vi "moveXYZ.vi"() -> ()   [LabVIEW 2014]
panel:
  in  "Z-Position":dbl=30.0
  in  "Y-Position":dbl
  in  "X-Position":dbl
  out "G-Code String":string
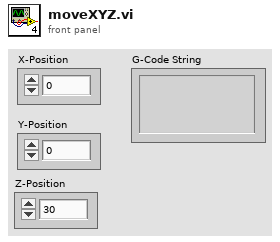
[diagram p1: front panel]
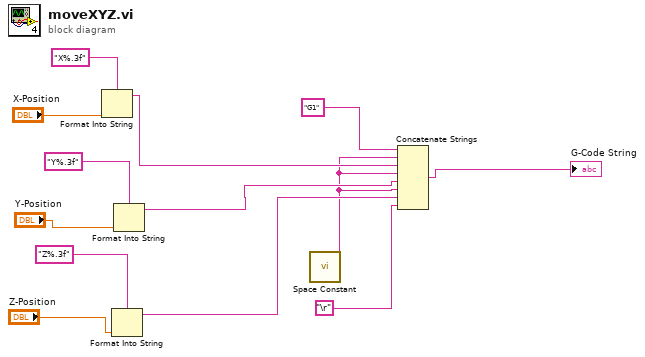
[diagram p0: block diagram]
diagram:
  n1 = Format Into String(format string="X%.3f", "X-Position") -> (resulting string=w7:string)  [unwired: 2 in, 1 out]
  n2 = Format Into String(format string="Z%.3f", "Z-Position") -> (resulting string=w5:string)  [unwired: 2 in, 1 out]
  n3 = Format Into String(format string="Y%.3f", "Y-Position") -> (resulting string=w6:string)  [unwired: 2 in, 1 out]
  n4 = call <vilib>:"Space Constant.vi"() -> ("String"=w3:string)
  n5 = Concatenate Strings("G1" ("string"), w3, w7, w3, w6, w3, w5, "\r") -> (→"G-Code String":string)
